vi "sequencerCWTopLevel.vi"() -> ()   [LabVIEW 2014]
uses:
  Controls/measVoltState.ctl
  sequencerState.ctl
  Controls/heinzingerSelect.ctl
  Controls/SPstate.ctl
  <vilib>/rvi/Emulation/niFpgaGetClockAttributes.vi
  <vilib>/rvi/Emulation/niFpgaSctlEmulationGetInTimedLoop.vi
  <vilib>/rvi/Emulation/niFpgaEmulationReportErrorSimple.vi
  sequencerGlobVars.vi
  MeasVolt/measVoltGlobVars.vi
  QueueHandler/queueHandlerGlobals.vi
  SimpleCounter/SCGlobVars.vi
  <vilib>/rvi/Emulation/niFpgaCriticalErrorInLSC.vi
panel:
  out "SPerrorCount":u8
  out "SPstate":T1
  in  "dwellTime":u32=2000000
  out "SPCtrQuWriteTimeout":bool
  in  "VoltOrScaler?":bool
  in  "stepSize":i32
  in  "start":i32
  in  "nOfSteps":i32
  in  "nOfScans":i32
  in  "invertScan":bool
  in  "heinzingerControl":T2=enum."Heinzinger0"
  in  "waitForKepco(25nsTicks)":u16
  in  "waitAfterReset(25nsTicks)":u16 caption="waitForDmm(25nsTicks)"
  in  "measVoltPulseLength(25ns)":i32
  in  "measVoltTimeout(10ns)":i32 caption="measVoltTimeout(25ns)"
  in  "timedOutWhileHandshake":bool
  out "seqState":T3
  in  "cmdByHost":T3
  in  "abort":bool
  in  "halt":bool
  in  "hostConfirmsHzOffsetIsSet":bool
  out "measVoltState":T4
  out "DACQuWriteTimeout":bool
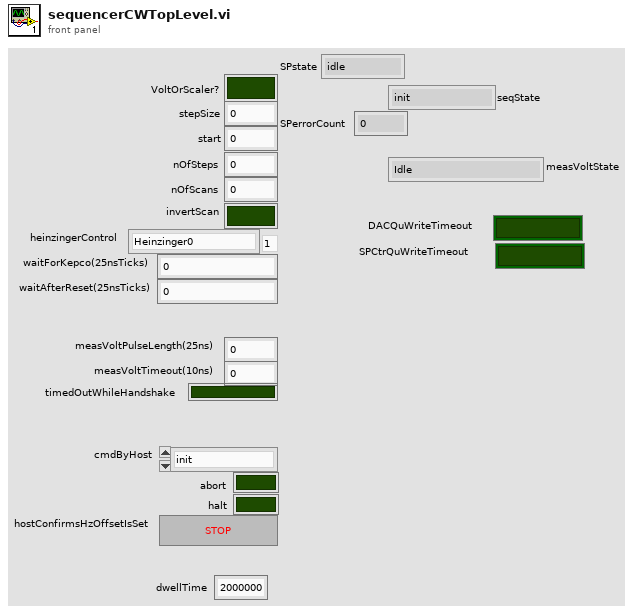
[diagram p1: front panel]
types:
  T1 = typedef "SPstate.ctl" = enum16{"idle", "scanning", "done", "error"}
  T2 = typedef "heinzingerSelect.ctl" = enum8{"Kepco", "Heinzinger0", "Heinzinger1", "Heinzinger2"}
  T3 = typedef "sequencerState.ctl" = enum16{"init", "idle", "measureOffset", "measureTrack", "measComplete", "error"}
  T4 = typedef "measVoltState.ctl" = enum16{"Idle", "sendMeasRequest", "waitUntilDone", "done"}
  T5 = cluster{"SCLK":refnum<k21>, "CS":refnum<k21>, "MOSI":refnum<k21>, "MISO":refnum<k21>}
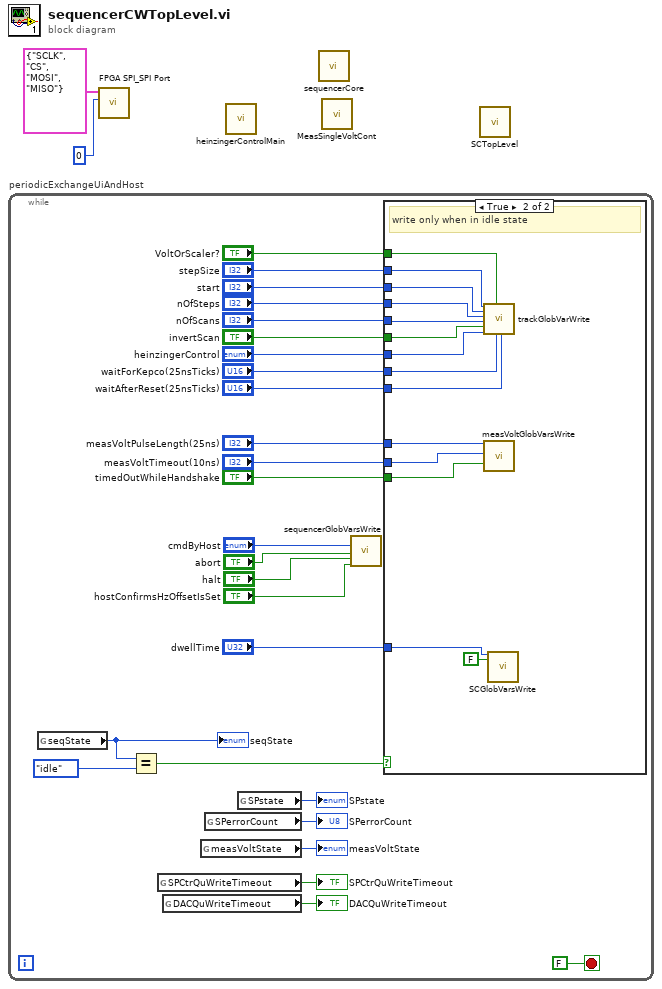
[diagram p0: block diagram]
diagram:
  n1 = while "periodicExchangeUiAndHost" {
    stop <- FALSE stop-if-true
    n2 = global read "sequencerGlobVars.vi" "seqState"() -> (w8:T3)
    "seqState" <- w8
    n3 = Equal?(x=w8, y=sequencerState."idle") -> (x = y?=w27:bool)
    n4 = global read "queueHandlerGlobals.vi" "SPCtrQuWriteTimeout"() -> (→"SPCtrQuWriteTimeout":bool)
    n5 = global read "queueHandlerGlobals.vi" "DACQuWriteTimeout"() -> (→"DACQuWriteTimeout":bool)
    n6 = global read "measVoltGlobVars.vi" "measVoltState"() -> (→"measVoltState":T4)
    n7 = global read "SCGlobVars.vi" "SPerrorCount"() -> (→"SPerrorCount":u8)
    n8 = global read "SCGlobVars.vi" "SPstate"() -> (→"SPstate":T1)
    n9 = call "sequencerGlobVarsWrite.vi"("cmdByHost"="cmdByHost", "abort"="abort", "halt"="halt", "hostConfirmsHzOffsetIsSet"="hostConfirmsHzOffsetIsSet") -> ()  [unwired: 16 in]
    n10 = case shown="True" w27 {
      tunnel: "VoltOrScaler?" -> [_ w42]
      tunnel: "stepSize" -> [_ w41]
      tunnel: "start" -> [_ w40]
      tunnel: "nOfSteps" -> [_ w39]
      tunnel: "nOfScans" -> [_ w38]
      tunnel: "invertScan" -> [_ w37]
      tunnel: "heinzingerControl" -> [_ w36]
      tunnel: "waitForKepco(25nsTicks)" -> [_ w35]
      tunnel: "waitAfterReset(25nsTicks)" -> [_ w34]
      tunnel: "measVoltPulseLength(25ns)" -> [_ w33]
      tunnel: "measVoltTimeout(10ns)" -> [_ w32]
      tunnel: "timedOutWhileHandshake" -> [_ w31]
      tunnel: "dwellTime" -> [_ w29]
      frame False {
      }
      frame True {
        # "write only when in idle state"
        n11 = call "trackGlobVarWrite.vi"("stepSize"=w41, "start"=w40, "nOfSteps"=w39, "nOfScans"=w38, "invertScan"=w37, "heinzingerControl"=w36, "VoltOrScaler?"=w42, "waitForKepco(25nsTicks)"=w35, "waitAfterReset(25nsTicks)"=w34) -> ()  [unwired: 11 in]
        n12 = call "measVoltGlobVarsWrite.vi"("measVoltPulseLength(25ns)"=w33, "measVoltTimeout(10ns)"=w32, "timedOutWhileHandshake"=w31) -> ()  [unwired: 17 in]
        n13 = call "SCGlobVarsWrite.vi"("dwellTime"=w29, "stop"=FALSE) -> ()  [unwired: 18 in]
      }
    }
  }
  n14 = call "FPGA SPI_SPI Port.vi"("Port"=i8 0, "FPGA IO"=T5 {"SCLK"="SCLK", "CS"="CS", "MOSI"="MOSI", "MISO"="MISO"}) -> ()  [unwired: 10 in]
  n15 = call "heinzingerControlMain.vi"() -> ()  [unwired: 3 in]
  n16 = call "sequencerCore.vi"() -> ()  [unwired: 12 in]
  n17 = call "MeasSingleVoltCont.vi"() -> ()  [unwired: 12 in]
  n18 = call "SCTopLevel.vi"() -> ()  [unwired: 12 in]
